vi "Normalise boolean maps to the longest length.vi"(8 "error in (no error)":errorcluster, 10 "Boolean Index map":refnum<class "2D Array binary.lvclass">, 11 "Line Profiles":refnum<class "2D Array f32.lvclass">) -> (0 "error out":errorcluster, 3 "Normalised Boolean Index Map":refnum<class "2D Array binary.lvclass">)   [LabVIEW 2020, in "G2CPU Line Profile.lvlib"]
uses:
  G2CPU Line Profile.lvlib
  <vilib>/Natan Biesmans/G2CPU GPU and CPU HPC Toolkit/G2CPU Libraries/Arrays/2DArray/f32/2D Array f32.lvclass
  C:/Program Files/National Instruments/LabVIEW 2025/vi.lib/Natan Biesmans/G2CPU GPU and CPU HPC Toolkit/G2CPU Libraries/Arrays/Array/Array Prototype.lvclass
  <vilib>/Natan Biesmans/G2CPU GPU and CPU HPC Toolkit/G2CPU Libraries/Arrays/2DArray/binary/2D Array binary.lvclass
  <vilib>/Natan Biesmans/G2CPU GPU and CPU HPC Toolkit/G2CPU Libraries/Arrays/Array/Array Prototype.lvclass/Array Prototype.ctl
  d7c48930-f628-4be5-b988-0aa312de1f48.vi
  66894469-523b-4234-a64e-0f23a6bbcd76.vi
  8f508d38-4889-46e3-8ec8-622df12fc188.vi
  bab79dbf-c22f-4f83-afdf-8e8e86bc3ad3.vi
  84d92f52-7e31-4259-94f3-60f3dca80432.vi
  bda65afe-89c5-426c-870a-75fa408a1887.vi
  6c602df9-ebce-4491-afa7-6f32799f5c3c.vi
  <vilib>/Natan Biesmans/G2CPU GPU and CPU HPC Toolkit/G2CPU Libraries/Arrays/Array/G2CPU Get Array Pointer.vi
  d7c48930-f628-4be5-b988-0aa312de1f48.vi/08cb2c43-1c8b-4a3a-83bc-b3e8cdef0e3a.vi
  d7c48930-f628-4be5-b988-0aa312de1f48.vi/6585f1b7-1f11-4b24-be38-c29351a5f24e.vi
  d7c48930-f628-4be5-b988-0aa312de1f48.vi/37397dd5-2c89-4701-b050-64d2f1e61e81.vi
  66894469-523b-4234-a64e-0f23a6bbcd76.vi/be773fc0-33da-4ff9-a1f3-1c8a600986f1.vi
  66894469-523b-4234-a64e-0f23a6bbcd76.vi/a8857c1c-6f29-49e3-99c3-b75749f7d80b.vi
  8f508d38-4889-46e3-8ec8-622df12fc188.vi/f4654d05-beb0-4753-bab7-24376daae318.vi
  8f508d38-4889-46e3-8ec8-622df12fc188.vi/a2f9e1c9-c94e-4cd6-9432-cf54c3ac582a.vi
  bab79dbf-c22f-4f83-afdf-8e8e86bc3ad3.vi/91a68f5e-71f7-47a4-9f0c-df2639fcd169.vi
  bab79dbf-c22f-4f83-afdf-8e8e86bc3ad3.vi/4a4570e6-0a54-4c17-842a-dba12dfc39a6.vi
  84d92f52-7e31-4259-94f3-60f3dca80432.vi/e7247370-a01f-465a-ac0e-4dfefcb1bb87.vi
  84d92f52-7e31-4259-94f3-60f3dca80432.vi/345e91f0-9a5e-4de4-af9c-133346717e4a.vi
  bda65afe-89c5-426c-870a-75fa408a1887.vi/492a4521-a697-4982-bdb9-a4b473f6765e.vi
  bda65afe-89c5-426c-870a-75fa408a1887.vi/b6d1f733-f67d-4708-929f-8d6c79a7c52f.vi
  6c602df9-ebce-4491-afa7-6f32799f5c3c.vi/80f98885-d133-4778-8a71-11569f5a634e.vi
  6c602df9-ebce-4491-afa7-6f32799f5c3c.vi/fede99c7-5d82-4ae2-b666-3731d213e31f.vi
  bab79dbf-c22f-4f83-afdf-8e8e86bc3ad3.vi/91a68f5e-71f7-47a4-9f0c-df2639fcd169.vi/edd31282-7992-4bba-af75-482693dee5e1.vi
  bda65afe-89c5-426c-870a-75fa408a1887.vi/b6d1f733-f67d-4708-929f-8d6c79a7c52f.vi/58bdfdf7-541c-4043-bcec-be03c1e23ff9.vi
  bda65afe-89c5-426c-870a-75fa408a1887.vi/b6d1f733-f67d-4708-929f-8d6c79a7c52f.vi/7af555d0-5c94-4227-839c-dec32778ebb2.vi
  6c602df9-ebce-4491-afa7-6f32799f5c3c.vi/80f98885-d133-4778-8a71-11569f5a634e.vi/6058dca8-195d-4566-b47b-6d6a1c5af61f.vi
  6c602df9-ebce-4491-afa7-6f32799f5c3c.vi/80f98885-d133-4778-8a71-11569f5a634e.vi/6058dca8-195d-4566-b47b-6d6a1c5af61f.vi/77c7badc-ed81-4514-99c1-20d37f4e5ecc.vi
  6c602df9-ebce-4491-afa7-6f32799f5c3c.vi/80f98885-d133-4778-8a71-11569f5a634e.vi/6058dca8-195d-4566-b47b-6d6a1c5af61f.vi/eb76fa01-6782-47b4-b34f-9eb474c9cc78.vi
  <vilib>/Natan Biesmans/G2CPU GPU and CPU HPC Toolkit/ArrayFire Driver/VIs/Run as Multi Device.vi
  <vilib>/Natan Biesmans/G2CPU GPU and CPU HPC Toolkit/G2CPU Libraries/Arrays/2DArray/s64/2D Array s64.lvclass
  <vilib>/Natan Biesmans/G2CPU GPU and CPU HPC Toolkit/ArrayFire Driver/VIs/diff1.vi
  <vilib>/Natan Biesmans/G2CPU GPU and CPU HPC Toolkit/G2CPU Libraries/Arrays/Array/G2CPU Set Array Pointer.vi
  <vilib>/Natan Biesmans/G2CPU GPU and CPU HPC Toolkit/G2CPU Libraries/Arrays/Array/G2CPU Release Array.vi
  <vilib>/Natan Biesmans/G2CPU GPU and CPU HPC Toolkit/ArrayFire Driver/VIs/isnan.vi
  <vilib>/Natan Biesmans/G2CPU GPU and CPU HPC Toolkit/ArrayFire Driver/VIs/not.vi
  <vilib>/Natan Biesmans/G2CPU GPU and CPU HPC Toolkit/ArrayFire Driver/VIs/and.vi
  <vilib>/Natan Biesmans/G2CPU GPU and CPU HPC Toolkit/ArrayFire Driver/VIs/cast.vi
  <vilib>/Natan Biesmans/G2CPU GPU and CPU HPC Toolkit/ArrayFire Driver/VIs/accum.vi
  <vilib>/Natan Biesmans/G2CPU GPU and CPU HPC Toolkit/G2CPU Libraries/Arrays/SubVI/RemoveReducedDimensionForReorder.vi
  <vilib>/Natan Biesmans/G2CPU GPU and CPU HPC Toolkit/ArrayFire Driver/VIs/reorder.vi
  <vilib>/Natan Biesmans/G2CPU GPU and CPU HPC Toolkit/ArrayFire Driver/VIs/release array.vi
  <vilib>/Natan Biesmans/G2CPU GPU and CPU HPC Toolkit/ArrayFire Driver/VIs/iszero.vi
  <vilib>/Natan Biesmans/G2CPU GPU and CPU HPC Toolkit/ArrayFire Driver/VIs/sub.vi
  <vilib>/Natan Biesmans/G2CPU GPU and CPU HPC Toolkit/ArrayFire Driver/subvi/Error Converter (ErrCode or Status).vi
  <vilib>/Natan Biesmans/G2CPU GPU and CPU HPC Toolkit/ArrayFire Driver/VIs/add.vi
  <vilib>/Natan Biesmans/G2CPU GPU and CPU HPC Toolkit/ArrayFire Driver/VIs/ge.vi
  <vilib>/Natan Biesmans/G2CPU GPU and CPU HPC Toolkit/G2CPU Libraries/Arrays/Array/Array Prototype.lvclass
  <vilib>/Natan Biesmans/G2CPU GPU and CPU HPC Toolkit/G2CPU Libraries/Arrays/DataTypes/f32/f32.lvclass
  <vilib>/Natan Biesmans/G2CPU GPU and CPU HPC Toolkit/G2CPU Libraries/Arrays/2DArray/2D Array Prototype.lvclass
  <vilib>/Natan Biesmans/G2CPU GPU and CPU HPC Toolkit/G2CPU Libraries/Arrays/DataTypes/I64/s64.lvclass
  <vilib>/Natan Biesmans/G2CPU GPU and CPU HPC Toolkit/G2CPU Libraries/Arrays/1DArray/s64/1D Array s64.lvclass
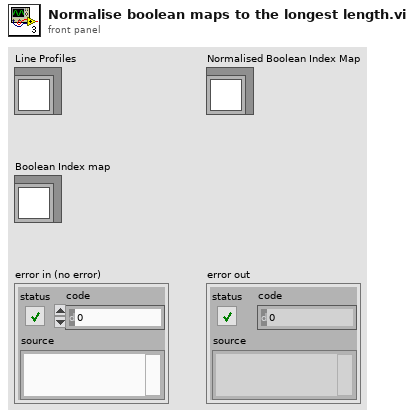
[diagram p1: front panel]
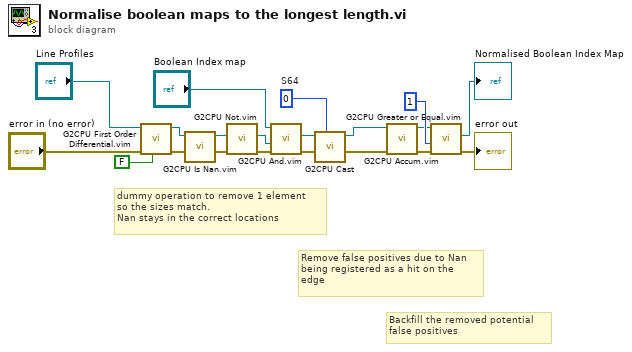
[diagram p0: block diagram]
diagram:
  w20 = i64 0  # S64
  # "Backfill the removed potential \nfalse positives"
  # "Remove false positives due to Nan\nbeing registered as a hit on the\nedge"
  # "dummy operation to remove 1 element\nso the sizes match.\nNan stays in the correct locations"
  n1 = call "G2CPU First Order Differential.vim"("Auto Release (Enabled)"=FALSE ("Auto Release Low (Enabled)"), "error in (no error)"="error in (no error)", "Array in"="Line Profiles") -> ("error out"=w13:errorcluster, "Array Result"=w12:refnum<class "2D Array f32.lvclass">)  [unwired: 7 in]
  n2 = call "G2CPU Is Nan.vim"("error in (no error)"=w13, "Array In"=w12) -> ("error out"=w9:errorcluster, "Array out"=w15:refnum<class "2D Array binary.lvclass">)  [unwired: 8 in]
  n3 = call "G2CPU Not.vim"("error in (no error)"=w9, "Array in"=w15) -> ("error out"=w8:errorcluster, "Array Result"=w10:refnum<class "2D Array binary.lvclass">)  [unwired: 8 in]
  n4 = call "G2CPU And.vim"("error in (no error)"=w8, "Array rhs"=w10, "Array lhs"="Boolean Index map") -> ("error out"=w16:errorcluster, "Array Result"=w17:refnum<class "2D Array binary.lvclass">)  [unwired: 7 in]
  n5 = call "G2CPU Cast"("Datatype Prototype"=w20, "error in (no error)"=w16, "Array In"=w17) -> ("error out"=w6:errorcluster, "Array Out"=w7:refnum<class "2D Array s64.lvclass">)  [unwired: 7 in]
  n6 = call "G2CPU Accum.vim"("error in (no error)"=w6, "Array in"=w7) -> ("error out"=w1:errorcluster, "Array Result"=w4:refnum<class "2D Array s64.lvclass">)  [unwired: 8 in]
  n7 = call "G2CPU Greater or Equal.vim"("error in (no error)"=w1, "Array rhs"=i64 1 ("Datatype Prototype"), "Array lhs"=w4) -> ("error out"=→"error out":errorcluster, "Array Result"=→"Normalised Boolean Index Map":refnum<class "2D Array binary.lvclass">)  [unwired: 7 in]
